vi "3.1-Arbitration Function.vi"() -> (0 "Motor Speed Setpoint (m/s)":dbl, 1 "Steering Angle Setpoint (deg)":dbl)   [LabVIEW 2010]
uses:
  3.0-Global.vi
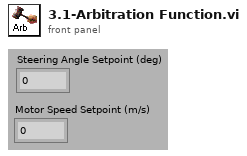
[diagram p1: front panel]
types:
  T1 = enum16{"Set Joystick", "Read Joystick", "Set Forebrain", "Read Forebrain", "Set Limbic", "Read Limbic", "Set Cerebellum", "Read Cerebellum", "Set Arbitrated", "Read Arbitrated", "Set LIDAR", "Read LIDAR"}
  T2 = typedef "4.1-Act Control Typedef.ctl" = cluster{"4.1.0 Data":string, "Type of Data":T3, "E-Stop":bool, "Restart":bool, "Extended Joystick":bool, "Begin":bool, "Time":i32, "Shutdown":bool}
  T3 = typedef "4.1.0-Datatype Typedef.ctl" = enum16{"4.1.0-Empty Data", "4.1.1-Joystick Data", "4.1.2-Behavioral Data"}
  T4 = typedef "4.1.2-Act Neuron TD.ctl" = cluster{"Speed By Path":dbl[]}
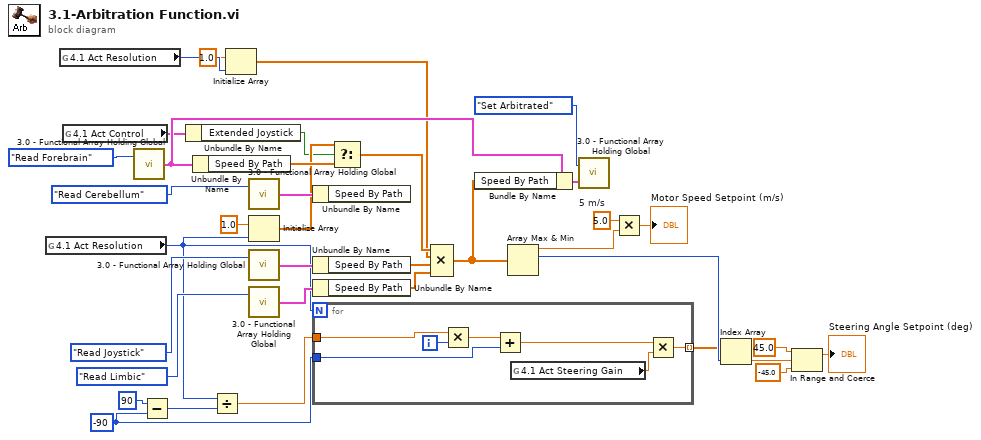
[diagram p0: block diagram]
diagram:
  w12 = -90 ("y")
  w32 = 5.0  # 5 m/s
  n1 = global read "3.0-Global.vi" "4.1 Act Resolution"() -> (w7:u32)
  n2 = global read "3.0-Global.vi" "4.1 Act Resolution"() -> (w3:u32)
  n3 = global read "3.0-Global.vi" "4.1 Act Control"() -> (w5:T2)
  n4 = call "3.0 - Functional Array Holding Global.vi"("Mode"=T1."Read Forebrain") -> ("Output Act Neurons"=w24:T4)  [unwired: 1 in]
  n5 = Subtract(x=90 ("y"), y=w12) -> (x-y=w14:i32)
  n6 = Unbundle By Name(w5) -> ("Extended Joystick"=w4:bool)
  n7 = Unbundle By Name(w24) -> ("Speed By Path"=w17:dbl[])
  n8 = Divide(x=w7, y=w14) -> (x/y=w13:dbl)
  n9 = Initialize Array(1.0 ("element"), w3) -> (w1:dbl[])
  n10 = call "3.0 - Functional Array Holding Global.vi"("Mode"=T1."Read Cerebellum") -> ("Output Act Neurons"=w22:T4)  [unwired: 1 in]
  n11 = Initialize Array(1.0 ("element"), w7) -> (w6:dbl[])
  n12 = call "3.0 - Functional Array Holding Global.vi"("Mode"=T1."Read Joystick") -> ("Output Act Neurons"=w23:T4)  [unwired: 1 in]
  n13 = call "3.0 - Functional Array Holding Global.vi"("Mode"=T1."Read Limbic") -> ("Output Act Neurons"=w25:T4)  [unwired: 1 in]
  n14 = Unbundle By Name(w22) -> ()  [unwired: 1 out]
  n15 = Unbundle By Name(w23) -> ("Speed By Path"=w20:dbl[])
  n16 = Unbundle By Name(w25) -> ("Speed By Path"=w19:dbl[])
  n17 = for {
    N: w7 -> [_]
    tunnel: [w38] -> w31 mode=indexing
    tunnel: w13 -> [w42]
    tunnel: w12 -> [w40]
    i -> [w39]
    n18 = Multiply(x=w42, y=w39) -> (x*y=w43:dbl)
    n19 = Add(x=w43, y=w40) -> (x+y=w41:dbl)
    n20 = global read "3.0-Global.vi" "4.1 Act Steering Gain"() -> (w37:dbl)
    n21 = Multiply(x=w41, y=w37) -> (x*y=w38:dbl)
  }
  n22 = Select(t=w6, s=w4, f=w17) -> (s? t:f=w16:dbl[])
  n23 = Compound Arithmetic op=MULTIPLY(w16, w1, w20, w19) -> (w18:dbl[])
  n24 = Bundle By Name(cluster=w24, "Speed By Path"=w18) -> (w21:T4)
  n25 = Array Max & Min(array=w18) -> (max value=w33:dbl, max index (indices)=w34:i32)  [unwired: 2 out]
  n26 = call "3.0 - Functional Array Holding Global.vi"("Input Act Neurons"=w21, "Mode"=T1."Set Arbitrated") -> ()  [unwired: 1 out]
  n27 = Multiply(x=w32, y=w33) -> (x*y=→"Motor Speed Setpoint (m/s)":dbl)
  n28 = Index Array(array=w31, index=w34) -> (element=w36:dbl)
  n29 = In Range and Coerce(upper limit=45.0, x=w36, lower limit=-45.0) -> (coerced(x)=→"Steering Angle Setpoint (deg)":dbl)  [unwired: 1 out]
